vi "SystemLink_Write_String.vi"(9 "String":string, 11 "SL_XControl":string(xcontrol)) -> ()   [LabVIEW 2020]
uses:
  SL_XControl.xctl
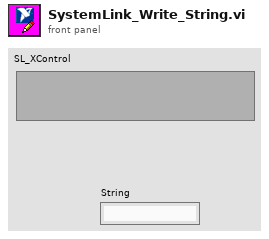
[diagram p1: front panel]
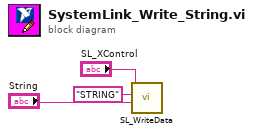
[diagram p0: block diagram]
diagram:
  n1 = call "SL_WriteData.vi"("Data"="String", "Type"="STRING", "Path"="SL_XControl") -> ()  [unwired: 9 in]
